vi "readFromXML.vi"(8 "error in (no error)":errorcluster, 10 "XML in":string="<MccTrack>\n <mccTrack>Off</mccTrack>\n</MccTrack>", 11 "MccTrack in":refnum<class "MccTrack.lvclass">) -> (0 "error out":errorcluster, 3 "MccTrack out":refnum<class "MccTrack.lvclass">)   [LabVIEW 2014, in "TCSDataDefinitions.lvlib" / "TCSMountControlCommand.lvlib" / "CommandsForAllAxes.lvlib" / "MccTrack.lvclass"]
uses:
  MccTrack.lvclass
  Enumerations/MountTrackStates.ctl
  MccTrack.lvclass/MccTrack.ctl
  CommandsForAllAxes.lvclass
  <userlib>/Common/XML/XMLParser/XMLParser.lvclass
  TCSMountControlCommand.lvlib
panel:
  out "data":T1=enum."Off"
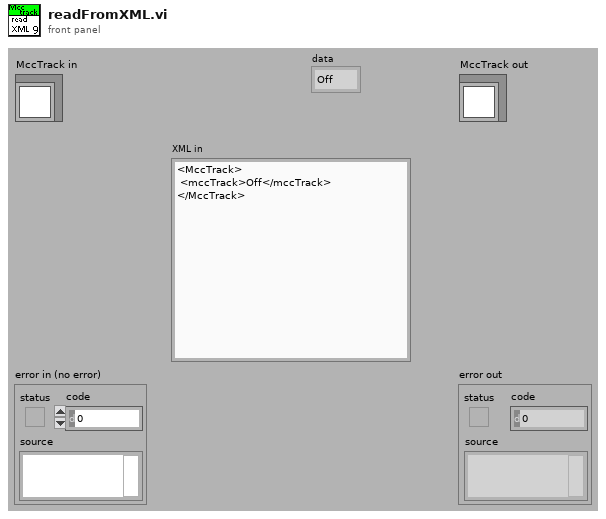
[diagram p1: front panel]
types:
  T1 = typedef "TCSDataDefinitions.lvlib/TCSMountControlCommand.lvlib/MountTrackStates.ctl" = enum16{"On", "Off"}
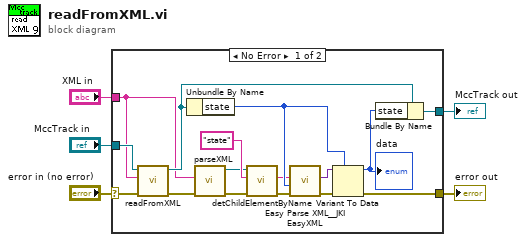
[diagram p0: block diagram]
diagram:
  n1 = case shown="No Error" "error in (no error)" {
    selector: "error in (no error)" -> [w13 w23]
    tunnel: [w16 w23] -> w4
    tunnel: [w17 w22] -> w2
    tunnel: "MccTrack in" -> [w15 w22]
    tunnel: "XML in" -> [w11 _]
    frame No Error {
      n2 = call-parent "readFromXML.vi"("error in (no error)"=w13, "XML in"=w11, "CommandsForAllAxes in"=w15) -> ("error out"=w10:errorcluster, "CommandsForAllAxes out"=w14:refnum<class "MccTrack.lvclass">)  [unwired: 7 out]
      n3 = Unbundle By Name(w14) -> ("state"=w19:T1)
      n4 = call <userlib>:"parseXML.vi"("error in (no error)"=w10, "XMLString in"=w11) -> ("error out"=w12:errorcluster, "Element out"=w6:refnum<class "XMLParser.lvclass">)  [unwired: 8 in]
      n5 = call <userlib>:"detChildElementByName.vi"("error in (no error)"=w12, "childName"="state" ("ChildName"), "Element in"=w6) -> ("error out"=w7:errorcluster, "childXML"=w8:string)  [unwired: 5 in, 2 out]
      n6 = call <vilib>:"Easy Parse XML__JKI EasyXML.vi"("error in (no error)"=w7, "LabVIEW Data (Type)"=w19, "XML String"=w8) -> ("error out"=w21:errorcluster, "LabVIEW Data"=w20:variant)  [unwired: 7 out]
      n7 = Variant To Data(error in=w21, type=w19, Variant=w20) -> (data=w18:T1, error out=w16:errorcluster)
      "data" <- w18
      n8 = Bundle By Name(cluster=w14, "state"=w18) -> (w17:refnum<class "MccTrack.lvclass">)
    }
    frame Error {
    }
  }
  "error out" <- w4
  "MccTrack out" <- w2
